vi "CommentFileHandler.vi"(8 "error in":errorcluster) -> (0 "error out":errorcluster)   [LabVIEW 2014]
uses:
  Controls/AddCommentParameters.ctl
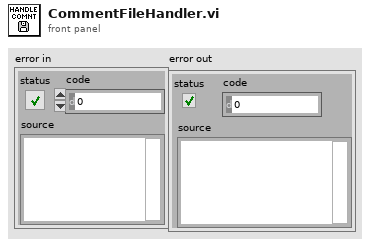
[diagram p1: front panel]
types:
  T1 = typedef "AddCommentParameters.ctl" = cluster{"PathConfig":path, "Comment":string}
  T2 = typedef "CommentLogClusterTypedef.ctl" = cluster{"variant":variant, "enum":T3}
  T3 = typedef "CommentLogEnumTypedef.ctl" = enum16{"AddComment", "Exit"}
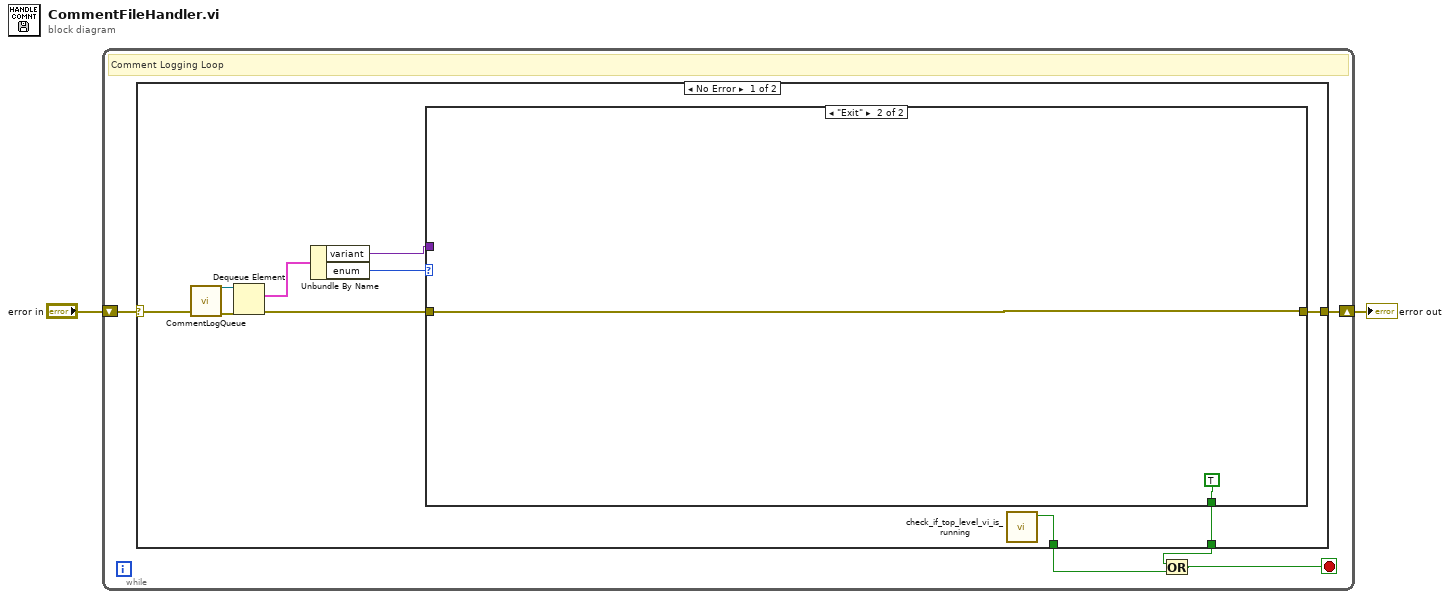
[diagram p0: block diagram]
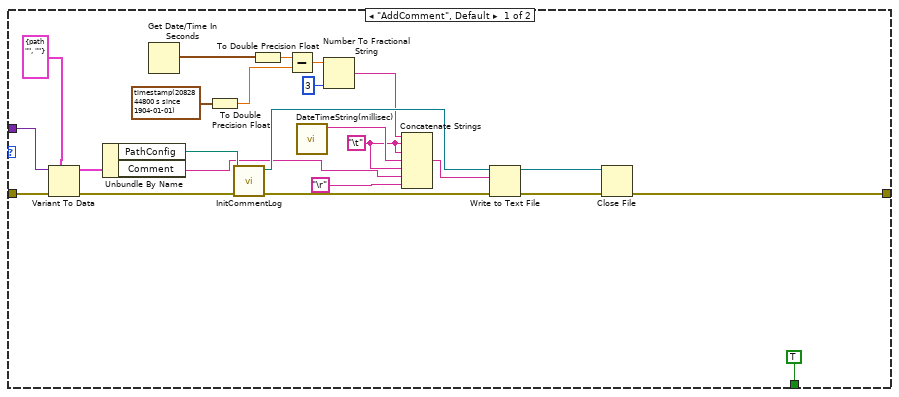
[diagram p2: hidden frame]
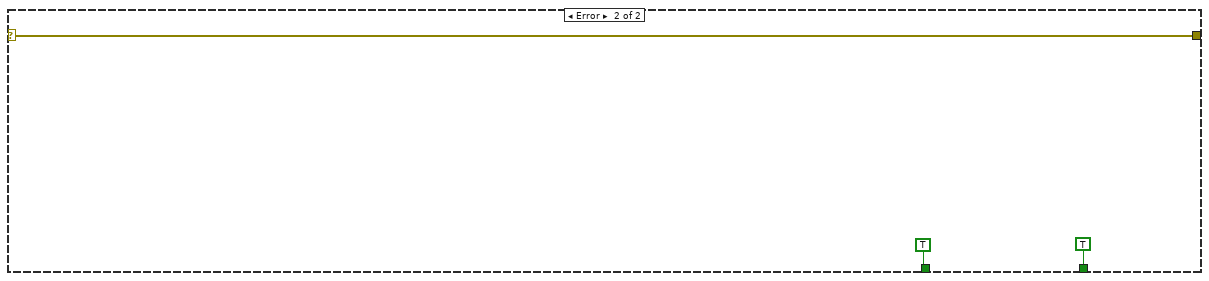
[diagram p3: hidden frame]
diagram:
  n1 = while {
    shift-right: [w7] -> w1
    shift-left: "error in" -> [w3]
    stop <- w6 stop-if-true
    # "Comment Logging Loop"
    n2 = case shown="No Error" w3 {
      selector: w3 -> [w8 w44]
      tunnel: [w13 w44] -> w7
      tunnel: [w10 TRUE] -> w5
      tunnel: [w9 TRUE ("stop?")] -> w4
      frame No Error {
        n3 = call "CommentLogQueue.vi"("error in"=w8) -> ("error out"=w11:errorcluster, "queue out"=w12:refnum<queue>)  [unwired: 8 in]
        n4 = Dequeue Element(queue=w12, error in (no error)=w11) -> (element=w17:T2, error out=w15:errorcluster)  [unwired: 1 in, 2 out]
        n5 = Unbundle By Name(w17) -> ("variant"=w14:variant, "enum"=w16:T3)
        n6 = case shown="\"Exit\"" w16 {
          tunnel: [w28 w43] -> w13
          tunnel: w15 -> [w40 w43]
          tunnel: [TRUE TRUE] -> w10
          tunnel: w14 -> [w41 _]
          frame "AddComment", Default {
            w33 = "\t"
            n7 = Variant To Data(error in=w40, type=T1 {"PathConfig"=path "", "Comment"=""}, Variant=w41) -> (data=w38:T1, error out=w39:errorcluster)
            n8 = Unbundle By Name(w38) -> ("PathConfig"=w37:path, "Comment"=w30:string)
            n9 = Get Date/Time In Seconds() -> (seconds since 1Jan1904=w22:timestamp)
            n10 = To Double Precision Float(number=timestamp(2082844800 s since 1904-01-01)) -> (double precision float=w24:dbl)
            n11 = call "InitCommentLog.vi"("error control"=w39, "file path (use dialog)"=w37) -> ("error indicator"=w32:errorcluster, "refnum out"=w31:refnum<file>)  [unwired: 8 in]
            n12 = To Double Precision Float(number=w22) -> (double precision float=w25:dbl)
            n13 = Subtract(x=w25, y=w24) -> (x-y=w21:dbl)
            n14 = call "DateTimeString(millisec).vi"() -> ("date/time string"=w34:string)  [unwired: 10 in, 1 out]
            n15 = Number To Fractional String(number=w21, precision (6)=i16 3) -> (F-format string=w20:string)  [unwired: 2 in]
            n16 = Concatenate Strings(w20, w33, w33, w34, w33, w30, "\r") -> (w36:string)
            n17 = Write to Text File(file (use dialog)=w31, text=w36, error in=w32) -> (refnum out=w27:refnum<file>, error out=w29:errorcluster)  [unwired: 1 in, 1 out]
            n18 = Close File(refnum=w27, error in=w29) -> (error out=w28:errorcluster)  [unwired: 1 out]
          }
          frame "Exit" {
          }
        }
        n19 = call "check_if_top_level_vi_is_running.vi"() -> ("stop?"=w9:bool)  [unwired: 10 in, 1 out]
      }
      frame Error {
      }
    }
    n20 = Or(x=w5, y=w4) -> (x .or. y?=w6:bool)
  }
  "error out" <- w1
